vi "API Test.vi"() -> ()   [LabVIEW 2016, in "Instrument.OxfordVRM.lvclass"]
uses:
  Instrument.OxfordVRM.lvclass
  Typedefs/Actions.ctl
  Typedefs/VRM Targets--Cluster.ctl
  Typedefs/Status.ctl
  <userlib>/LevyLab/Levylab Instruments/Instrument Types/Cryostat/Typedefs/VRM Magnet Axis--Enum.ctl
panel:
  out "Actions 2":T1
  out "Status":T2
  in  "Targets":T3
  in  "Actions":T1
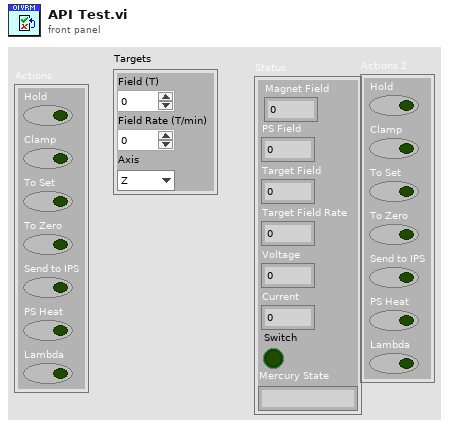
[diagram p1: front panel]
types:
  T1 = typedef "Instrument.OxfordVRM.lvclass/Actions.ctl" = cluster{"Hold":bool, "Clamp":bool, "To Set":bool, "To Zero":bool, "Send to IPS":bool, "PS Heat":bool, "Lambda":bool}
  T2 = typedef "Instrument.OxfordVRM.lvclass/Status.ctl" = cluster{"Magnet Field":dbl, "PS Field":dbl, "Target Field":dbl, "Target Field Rate":dbl, "Voltage":dbl, "Current":dbl, "Switch":bool, "Mercury State":string}
  T3 = typedef "Instrument.OxfordVRM.lvclass/VRM Targets--Cluster.ctl" = cluster{"Field (T)":dbl, "Field Rate (T/min)":dbl, "Axis":T4}
  T4 = typedef "Instrument.OxfordVRM.lvclass/VRM Magnet Axis--Enum.ctl" = enum16{"Z", "X", "Y", "ALL"}
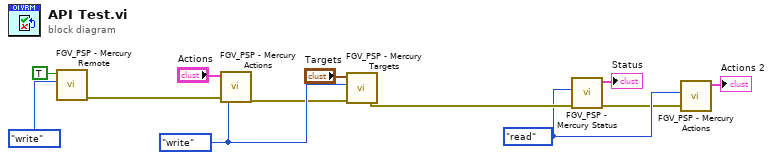
[diagram p0: block diagram]
diagram:
  w3 = enum16{"write", "read"}."read" ("Function")
  w8 = enum16{"write", "read"}."write" ("Function")
  n1 = call "FGV_PSP - Mercury Remote.vi"("Function"=enum16{"write", "read"}."write", "Remote"=TRUE) -> ("error out"=w11:errorcluster)  [unwired: 4 in, 1 out]
  n2 = call "FGV_PSP - Mercury Actions.vi"("error in"=w11, "Function"=w8, "Actions"="Actions") -> ("error out"=w6:errorcluster)  [unwired: 3 in, 1 out]
  n3 = call "FGV_PSP - Mercury Targets.vi"("error in"=w6, "Function"=w8, "Targets"="Targets") -> ("error out"=w5:errorcluster)  [unwired: 3 in, 1 out]
  n4 = call "FGV_PSP - Mercury Status.vi"("error in"=w5, "Function"=w3) -> ("error out"=w2:errorcluster, "Status"=→"Status":T2)  [unwired: 4 in]
  n5 = call "FGV_PSP - Mercury Actions.vi"("error in"=w2, "Function"=w3) -> ("Actions"=→"Actions 2":T1)  [unwired: 4 in, 1 out]
